vi "Basic Example.vi"() -> ()   [LabVIEW 2016, in "LIFA MPU-60X0.lvlib"]
uses:
  LIFA MPU-60X0.lvlib
  DeviceAddresses.ctl
panel:
  in  "Stop Button":bool
  out "Temperature (°C)":dbl(slide) scale=0.0..100.0
  out "Gyro Data":T1(graph)
  out "Accelerometer Data":T1(graph)
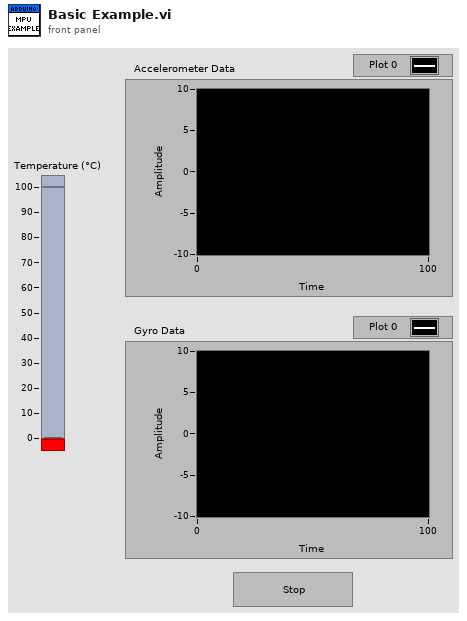
[diagram p1: front panel]
types:
  T1 = cluster{"X-axis":i16, "Y-axis":i16, "Z-axis":i16}
  T2 = typedef "LIFA MPU-60X0.lvlib/DeviceAddresses.ctl" = u8
  T3 = typedef "LabVIEW Interface for Arduino.lvlib/Arduino Resource.ctl" = cluster{"VISA resource":refnum<visa-resource-name>, "Board Type":T4, "Connection Type":enum8{"USB / Serial"}, "Bytes Per Packet (15)":u8}
  T4 = typedef "LabVIEW Interface for Arduino.lvlib/Board Type.ctl" = enum16{"Uno", "Dimuelanove w/Atmega 328", "Mega 2560"}
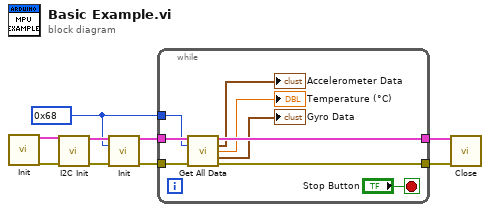
[diagram p0: block diagram]
diagram:
  w3 = T2 104 items=["0x68"=104, "0x69"=105] ("Device Address")
  n1 = call <vilib>:"Init.vi"() -> ("Arduino Resource"=w5:T3, "error out"=w4:errorcluster)  [unwired: 18 in]
  n2 = call <vilib>:"I2C Init.vi"("Arduino Resource"=w5, "error in"=w4) -> ("Arduino Resource"=w9:T3, "error out"=w8:errorcluster)  [unwired: 12 in]
  n3 = call <vilib>:"Init.vi"("Arduino Resource"=w9, "Device Address"=w3, "error in (no error)"=w8) -> ("Arduino Resource"=w7:T3, "error out"=w6:errorcluster)  [unwired: 11 in]
  n4 = while {
    tunnel: w7 -> [w18]
    tunnel: w6 -> [w17]
    tunnel: w3 -> [w16]
    tunnel: [w15] -> w2
    tunnel: [w14] -> w1
    stop <- "Stop Button" stop-if-true
    n5 = call "Get All Data.vi"("Arduino Resource"=w18, "Device Address"=w16, "error in (no error)"=w17) -> ("Arduino Resource"=w15:T3, "Accel Data"=→"Accelerometer Data":T1, "Temperature (°C)"=→"Temperature (°C)":dbl, "Gyro Data"=→"Gyro Data":T1, "error out"=w14:errorcluster)  [unwired: 8 in]
  }
  n6 = call <vilib>:"Close.vi"("Arduino Resource"=w2, "error in"=w1) -> ()  [unwired: 13 in, 1 out]
